vi "Analyse_Error.vi"(0 "Erroe_Under_Analyse":errorcluster, 11 "Error_In":errorcluster) -> (4 "State_and_Data":T1, 15 "Error_Out":errorcluster)   [LabVIEW 2021]
doc: "Used to analyse the error"
uses:
  Controls/State_and_Data.ctl
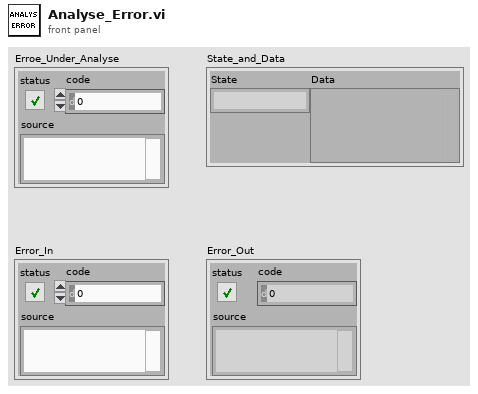
[diagram p1: front panel]
types:
  T1 = typedef "State_and_Data.ctl" = cluster{"State":string, "Data":variant}
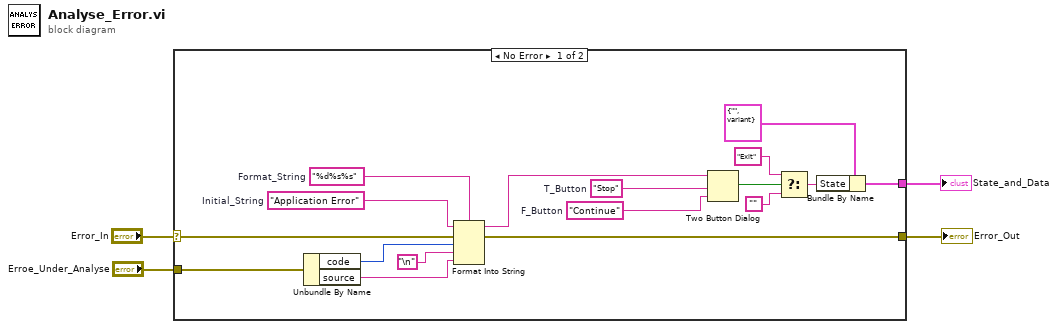
[diagram p0: block diagram]
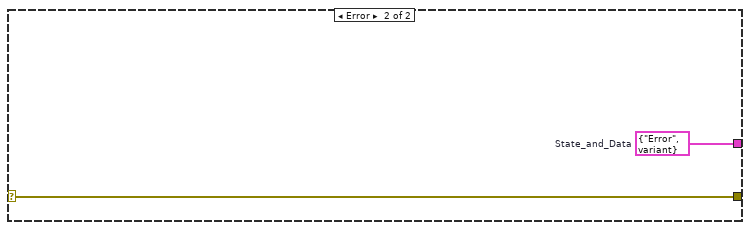
[diagram p2: hidden frame]
diagram:
  n1 = case shown="No Error" "Error_In" {
    selector: "Error_In" -> [w9 w23]
    tunnel: [w8 w23] -> w2
    tunnel: "Erroe_Under_Analyse" -> [w7 _]
    tunnel: [w5 w22] -> w4
    frame No Error {
      w17 = "%d%s%s"  # Format_String
      w18 = "Application Error"  # Initial_String
      w19 = "Stop"  # T_Button
      w20 = "Continue"  # F_Button
      n2 = Unbundle By Name(w7) -> ("code"=w15:i32, "source"=w14:string)
      n3 = Format Into String(format string=w17, initial string=w18, error in=w9, w15, "\n", w14) -> (resulting string=w21:string, error out=w8:errorcluster)
      n4 = Two Button Dialog(message=w21, 1:w20, 2:w19) -> (T button?=w12:bool)
      n5 = Select(t="Exit" ("State"), s=w12, f="") -> (s? t:f=w10:string)
      n6 = Bundle By Name(cluster=T1 {"State"="", "Data"=variant} ("State_and_Data"), "State"=w10) -> (w5:T1)
    }
    frame Error {
      w22 = T1 {"State"="Error", "Data"=variant}  # State_and_Data
    }
  }
  "State_and_Data" <- w4
  "Error_Out" <- w2
